vi "Get Resource ID.vi"(4 "I2C in":refnum<class "I2C.lvclass">) -> (7 "Resource ID":string)   [LabVIEW 2024, in "CTI.lvlib" / "I2C.lvclass"]
uses:
  I2C.lvclass
  I2C.lvclass/I2C.ctl
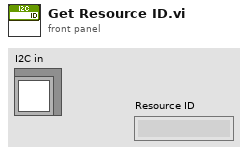
[diagram p1: front panel]
types:
  T1 = typedef "CTI.lvlib/I2C Number.ctl" = i8
  T2 = typedef "CTI.lvlib/GPIO Number.ctl" = i8
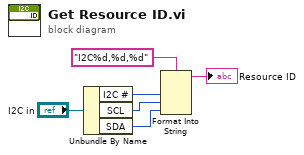
[diagram p0: block diagram]
diagram:
  n1 = Unbundle By Name("I2C in") -> ("I2C #"=w2:T1, "SCL"=w4:T2, "SDA"=w3:T2)
  n2 = Format Into String(format string="I2C%d,%d,%d", w2, w4, w3) -> (resulting string=→"Resource ID":string)  [unwired: 2 in, 1 out]
